vi "Swapit2D (SubVI).vi"(1 "oriplot":dbl[][](array[numeric])) -> (0 "Zero-centerd Xcor":dbl[][](graph))   [LabVIEW 2011, in "OfflineTracker.lvlib"]
uses:
  OfflineTracker.lvlib
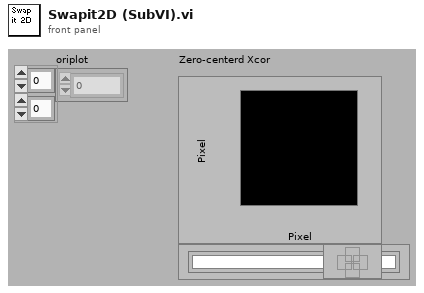
[diagram p1: front panel]
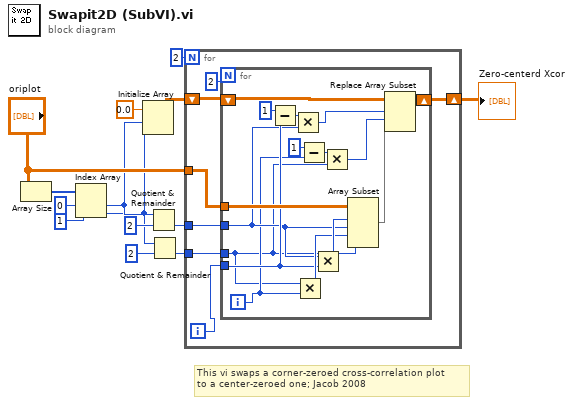
[diagram p0: block diagram]
diagram:
  # "This vi swaps a corner-zeroed cross-correlation plot\nto a center-zeroed one; Jacob 2008"
  n1 = Array Size(array="oriplot") -> (size(s)=w9:i32[])
  n2 = Index Array(array=w9, index #1=0 ("index"), index #2=1 ("index")) -> (element #1=w8:i32, element #2=w7:i32)
  n3 = Initialize Array(0.0 ("element"), w8, w7) -> (w2:dbl[][])
  n4 = Quotient & Remainder(x=w8, y=2) -> (floor(x/y)=w5:i32)  [unwired: 1 out]
  n5 = Quotient & Remainder(x=w7, y=2) -> (floor(x/y)=w4:i32)  [unwired: 1 out]
  n6 = for {
    N: 2 -> [_]
    tunnel: "oriplot" -> [w21]
    tunnel: w5 -> [w20]
    tunnel: w4 -> [w19]
    shift-right: [w15] -> w1
    shift-left: w2 -> [w16]
    i -> [w18]
    n7 = for {
      N: 2 -> [_]
      tunnel: w21 -> [w37]
      tunnel: w20 -> [w28]
      tunnel: w19 -> [w23]
      tunnel: w18 -> [w30]
      shift-right: [w32] -> w15
      shift-left: w16 -> [w34]
      i -> [w24]
      n8 = Subtract(x=u32 1, y=w30) -> (x-y=w29:u32)
      n9 = Multiply(x=w29, y=w28) -> (x*y=w27:u32)
      n10 = Multiply(x=w23, y=w24) -> (x*y=w35:i32)
      n11 = Subtract(x=u32 1, y=w24) -> (x-y=w25:u32)
      n12 = Multiply(x=w28, y=w30) -> (x*y=w36:i32)
      n13 = Multiply(x=w25, y=w23) -> (x*y=w22:u32)
      n14 = Array Subset(array=w37, index (row)=w36, length (row)=w28, index (col)=w35, length (col)=w23) -> (w33:dbl[][])
      n15 = Replace Array Subset(array=w34, new element=w33, index (row)=w27, index (col)=w22) -> (w32:dbl[][])
    }
  }
  "Zero-centerd Xcor" <- w1
